vi "Write Client ID.vi"(8 "error in (no error)":errorcluster, 10 "Client ID":string, 11 "Oauth2 in":refnum<class "Oauth2.lvclass">) -> (0 "error out":errorcluster, 3 "Oauth2 out":refnum<class "Oauth2.lvclass">)   [LabVIEW 2013, in "Oauth2.lvclass"]
uses:
  Oauth2.lvclass
  Oauth2.lvclass/Oauth2.ctl
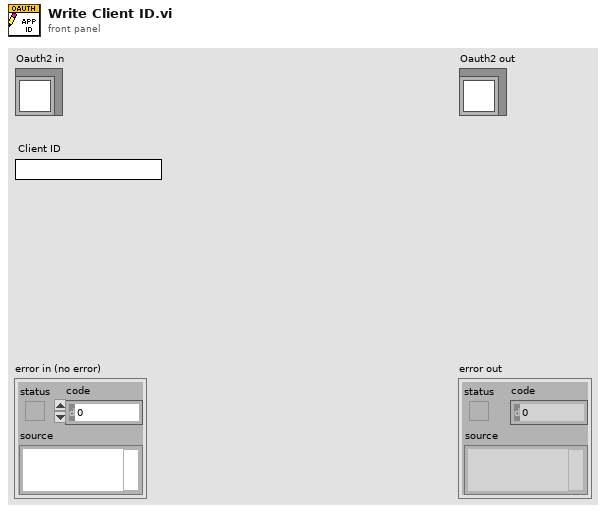
[diagram p1: front panel]
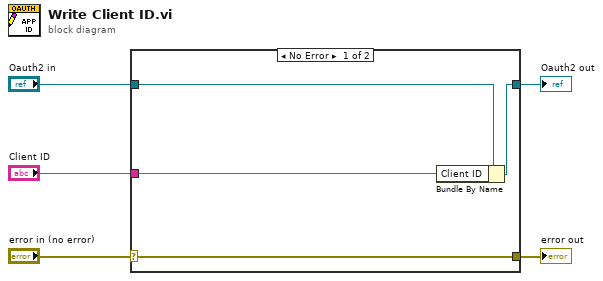
[diagram p0: block diagram]
diagram:
  n1 = case shown="No Error" "error in (no error)" {
    selector: "error in (no error)" -> [w9 w10]
    tunnel: [w9 w10] -> w4
    tunnel: [w7 w11] -> w2
    tunnel: "Oauth2 in" -> [w8 w11]
    tunnel: "Client ID" -> [w6 _]
    frame No Error {
      n2 = Bundle By Name(cluster=w8, "Client ID"=w6) -> (w7:refnum<class "Oauth2.lvclass">)
    }
    frame Error {
    }
  }
  "error out" <- w4
  "Oauth2 out" <- w2
